vi "Dead Ban.vi"(1 "Joy IN":dbl) -> (0 "Joy OUT":dbl)   [LabVIEW 2013]
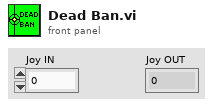
[diagram p1: front panel]
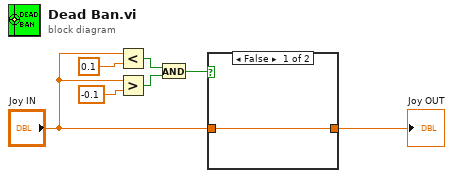
[diagram p0: block diagram]
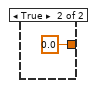
[diagram p2: hidden frame]
diagram:
  n1 = Less?(x="Joy IN", y=0.1) -> (x < y?=w6:bool)
  n2 = Greater?(x="Joy IN", y=-0.1) -> (0:w7:bool)
  n3 = And(x=w6, y=w7) -> (x .and. y?=w3:bool)
  n4 = case shown="False" w3 {
    tunnel: [w8 0.0 ("Joy IN")] -> w2
    tunnel: "Joy IN" -> [w8 _]
    frame False {
    }
    frame True {
    }
  }
  "Joy OUT" <- w2
